vi "super small oscilloscope.vi"() -> ()   [LabVIEW 2017]
uses:
  <vilib>/Instr/_visa.llb/VISA Set IO Buffer Mask.ctl
  typedefs/reading3.ctl
  <vilib>/Platform/TimedLoop/XDataNode/timing_clust.ctl
  <vilib>/Platform/TimedLoop/XDataNode/nitl_modes.ctl
  <vilib>/Platform/TimedLoop/XDataNode/wakeup.ctl
  typedefs/reading1.ctl
  <vilib>/Analysis/6fits.llb/Curve Fitting Criteria.ctl
  <vilib>/Analysis/baseanly.llb/Mean (DBL).vi
  <vilib>/Instr/_visa.llb/VISA Configure Serial Port (Instr).vi
  <vilib>/platform/TimedLoop/XDataNode/XDataNode.xnode
  <vilib>/Platform/TimedLoop/XDataNode/XDNodeRunTimeDep.lvlib
  <vilib>/Analysis/NI_AALPro.lvlib
  <vilib>/ptbypt/NI_PtbyPt.lvlib
  <vilib>/Analysis/NI_AALBase.lvlib
panel:
  out "z accel":dbl format="%0.2f"
  out "Yaccel":dbl(slide) scale=-1.0..1.0
  out "Xaccel":dbl(slide) scale=-1.0..1.0
  in  "rest":bool
  out "error":i32
  out "deg/hr":dbl format="%0.2f"
  out "Waveform Chart":dbl(graph)
  out "angle":dbl
  out "slope":dbl
  out "magnet":cluster{dbl[], "Best Linear Fit":dbl[]}[](graph)
  in  "time range (s)":dbl=2.2 format="%#_13g"
  in  "stop 2":bool
  out "voltage":cluster{dbl[], dbl[]}[](graph)
  in  "update (ms)":i64=100
  out "error out":errorcluster
  in  "stop":bool
  in  "VISA resource name":refnum<visa-resource-name>
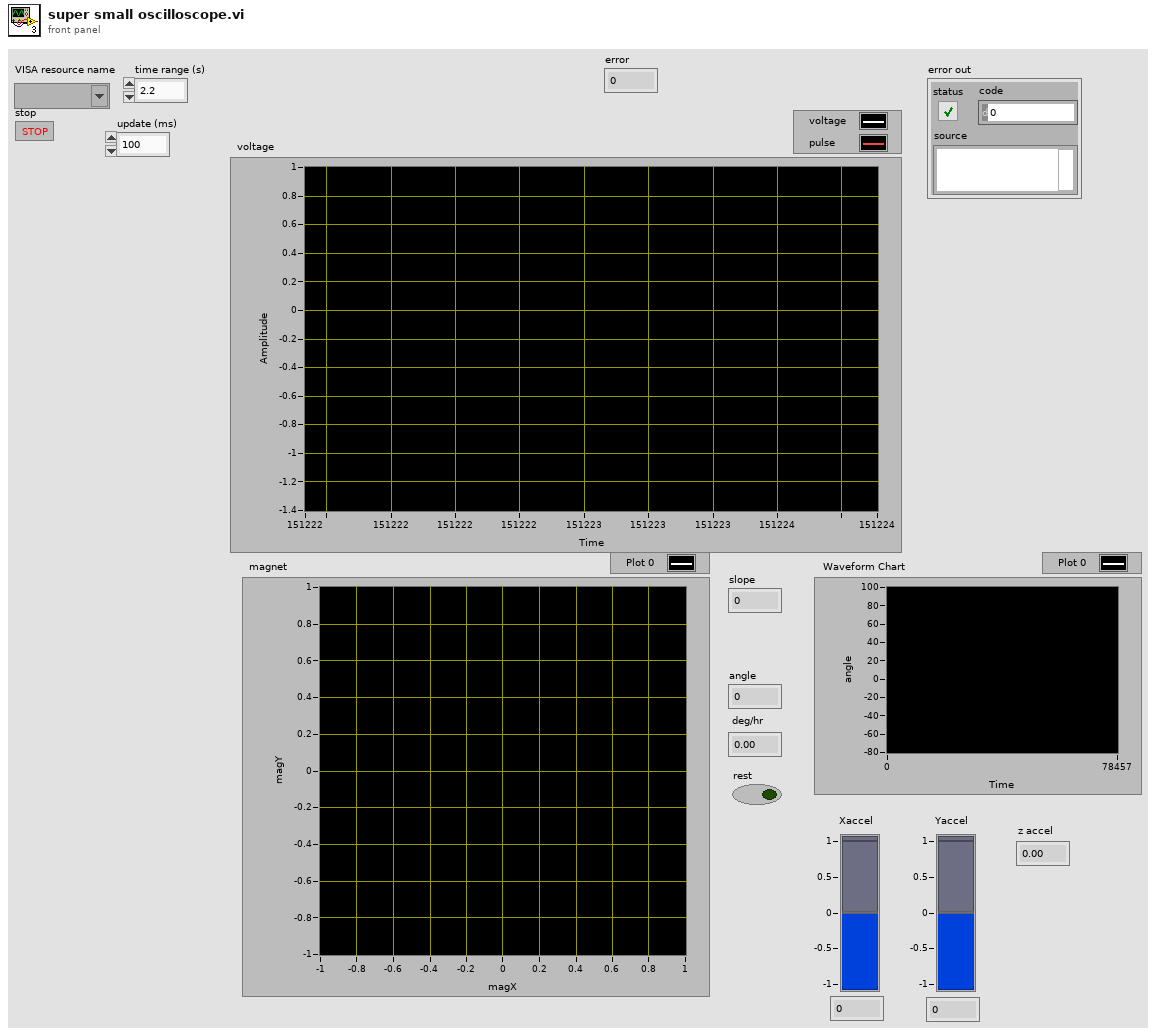
[diagram p1: front panel]
types:
  T1 = typedef "reading3.ctl" = cluster{"time":dbl, "x":dbl, "y":dbl, "z":dbl}
  T2 = typedef "VISA Set IO Buffer Mask.ctl" = u16
  T3 = typedef "reading1.ctl" = cluster{"time":dbl, "x":dbl}
  T4 = typedef "XDNodeRunTimeDep.lvlib/timing_clust.ctl" = cluster{"Expected End [f-1]":u64, "Actual End [f-1]":u64, "Finished Late? [f-1]":bool, "Expected End [i-1]":u64, "Actual End [i-1]":u64, "Finished Late? [i-1]":bool, "Expected Start [i]":u64, "Actual Start [i]":u64, "Expected Start [f]":u64, "Actual Start [f]":u64, "Source Name":string, "Structure Name":string, "Period":i64, "Deadline":i64, "Offset":i64, "Start":i64, "Priority":i32, "Timeout":i32, "Mode":T5, "Wakeup Reason":T6, "Error":errorcluster, "Source Type":string, "Secondary Source Type":string, "Global End Time":u64, "Global Start Time":u64, "Frame Duration":u64, "Iteration Duration":u64, "Assigned CPU":i32, "I/O Scan Engine Mode":u32}
  T5 = typedef "XDNodeRunTimeDep.lvlib/nitl_modes.ctl" = enum32{"No Change", "Process missed periods, maintain original phase", "Discard missed periods, maintain original phase", "Process missed periods, ignore original phase", "Discard missed periods, ignore original phase"}
  T6 = typedef "XDNodeRunTimeDep.lvlib/wakeup.ctl" = enum32{"Normal", "Aborted", "Asynchronous wakeup", "Timing source error", "Timed loop error", "Timeout"}
  T7 = typedef "NI_AALPro.lvlib/Curve Fitting Criteria.ctl" = u16
  T8 = cluster{"Best Linear Fit":dbl[], "Best Linear Fit":dbl[]}
  T9 = cluster{"Best Linear Fit":dbl[], "Best Linear Fit":dbl[]}[]
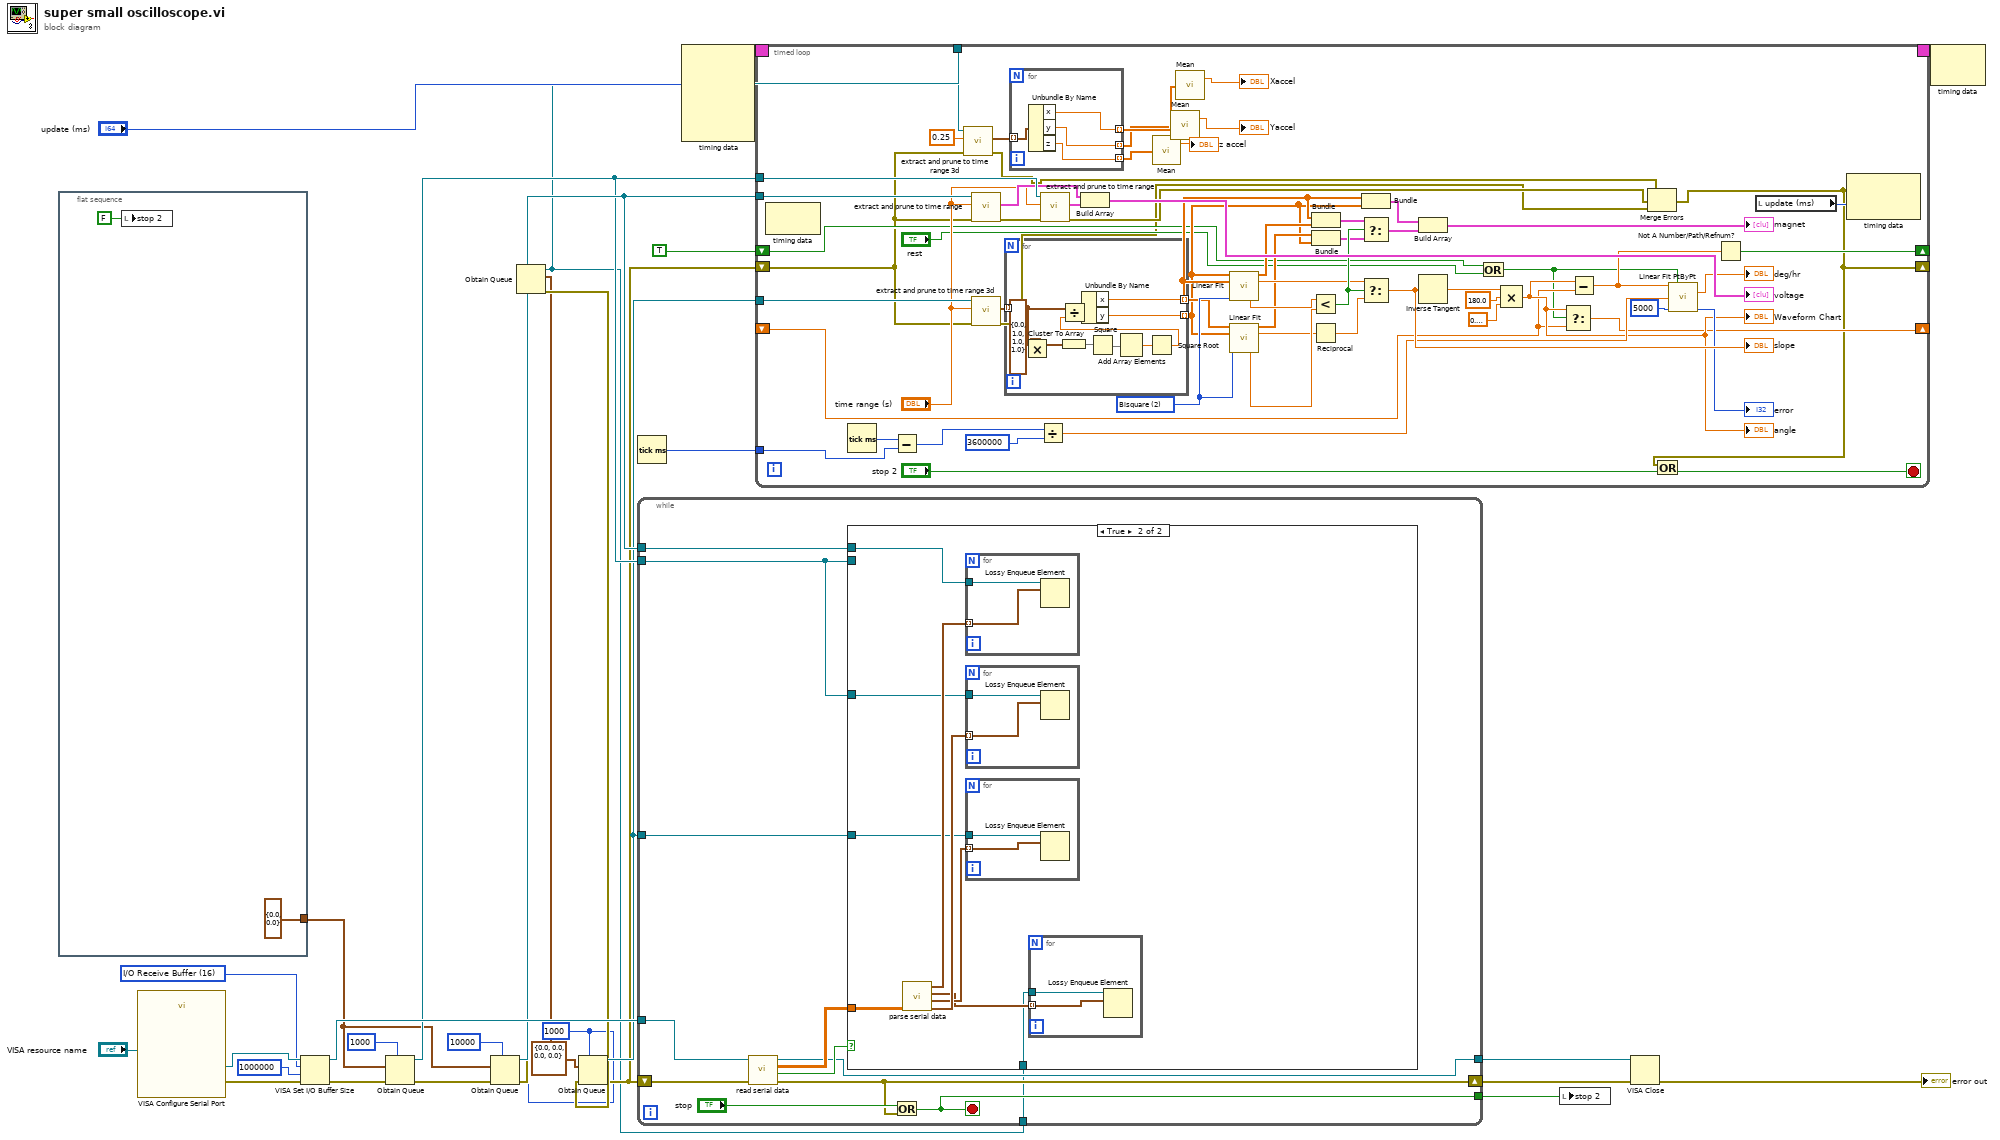
[diagram p0: block diagram]
diagram:
  w2 = 1000 ("max queue size (-1, unlimited)")
  w3 = T1 {"time"=0.0, "x"=0.0, "y"=0.0, "z"=0.0} ("reading3")
  w25 = T2 16 items=["I/O Receive Buffer"=16, "I/O Transmit Buffer"=32, "I/O Receive and Transmit Buffer"=48] ("Mask")
  n1 = flat-sequence {
    tunnel: [T3 {"time"=0.0, "x"=0.0} ("reading1")] -> w14
    frame #0 {
      n2 = local write "stop 2"(FALSE ("stop 2")) -> ()
    }
  }
  n3 = call-poly "VISA Configure Serial Port"("VISA resource name"="VISA resource name") -> ("VISA resource name out"=w28:refnum<visa-resource-name>, "error out"=w24:errorcluster)  [unwired: 13 in]
  n4 = VISA Set I/O Buffer Size(VISA resource name=w28, mask (16)=w25, size (4096)=u32 1000000, error in (no error)=w24) -> (VISA resource name out=w27:refnum<visa-resource-name>, error out=w17:errorcluster)
  n5 = Obtain Queue(max queue size (-1, unlimited)=1000, element data type=w14, error in (no error)=w17) -> (queue out=w15:refnum<queue>, error out=w13:errorcluster)  [unwired: 2 in, 1 out]
  n6 = Obtain Queue(max queue size (-1, unlimited)=10000, element data type=w14, error in (no error)=w13) -> (queue out=w19:refnum<queue>, error out=w6:errorcluster)  [unwired: 2 in, 1 out]
  n7 = Obtain Queue(max queue size (-1, unlimited)=w2, element data type=w3, error in (no error)=w6) -> (queue out=w1:refnum<queue>, error out=w5:errorcluster)  [unwired: 2 in, 1 out]
  n8 = Obtain Queue(max queue size (-1, unlimited)=w2, element data type=w3, error in (no error)=w5) -> (queue out=w9:refnum<queue>, error out=w4:errorcluster)  [unwired: 2 in, 1 out]
  n9 = Tick Count (ms)() -> (millisecond timer value=w8:u32)
  n10 = while {
    tunnel: w27 -> [w42]
    shift-right: [w38] -> w11
    shift-left: w4 -> [w41]
    tunnel: w19 -> [w37]
    tunnel: [w36] -> w18
    tunnel: w15 -> [w35]
    tunnel: [w34] -> w12
    tunnel: w9 -> [w33]
    tunnel: w1 -> [w32]
    stop <- w36 stop-if-true
    n11 = call "read serial data.vi"("error in (no error)"=w41, "serial port"=w42) -> ("error out"=w38:errorcluster, "data read"=w39:bool, "serial data"=w40:dbl[][], "VISA resource name out"=w34:refnum<visa-resource-name>)  [unwired: 6 in]
    n12 = case shown="True" w39 {
      tunnel: w40 -> [_ w52]
      tunnel: w37 -> [_ w50]
      tunnel: w35 -> [_ _]
      tunnel: w35 -> [_ w49]
      tunnel: w33 -> [_ w46]
      tunnel: w32 -> [_ w44]
      frame False {
      }
      frame True {
        n13 = call "parse serial data.vi"("serial data"=w52) -> ("coil data"=w48:T3[], "mag data"=w47:T1[], "accel data"=w45:T1[], "voltage data"=w51:T3[])  [unwired: 7 in]
        n14 = for {
          tunnel: w51 -> [w59] mode=indexing
          tunnel: w50 -> [w60]
          n15 = Lossy Enqueue Element(queue=w60, element=w59) -> ()  [unwired: 1 in, 4 out]
        }
        n16 = for {
          tunnel: w49 -> [w58]
          tunnel: w48 -> [w57] mode=indexing
          n17 = Lossy Enqueue Element(queue=w58, element=w57) -> ()  [unwired: 1 in, 4 out]
        }
        n18 = for {
          tunnel: w47 -> [w56] mode=indexing
          tunnel: w46 -> [w55]
          n19 = Lossy Enqueue Element(queue=w55, element=w56) -> ()  [unwired: 1 in, 4 out]
        }
        n20 = for {
          tunnel: w45 -> [w54] mode=indexing
          tunnel: w44 -> [w53]
          n21 = Lossy Enqueue Element(queue=w53, element=w54) -> ()  [unwired: 1 in, 4 out]
        }
      }
    }
    n22 = Or(x="stop", y=w38) -> (x .or. y?=w36:bool)
  }
  n23 = node-c288("update (ms)") -> (w22:T4)  [unwired: 4 in]
  n24 = timed-loop {
    timing: w22 -> [_]
    timing-out: [_] -> w21
    tunnel: w19 -> [w119]
    tunnel: w15 -> [w117]
    tunnel: w9 -> [w114]
    tunnel: w8 -> [w89]
    shift-right: [w83] -> _
    shift-left: _ -> [w82]
    shift-right: [w80] -> _
    shift-left: TRUE -> [w79]
    shift-right: [w72] -> _
    shift-left: w4 -> [w62]
    tunnel: w1 -> [w70]
    stop <- w73 stop-if-true
    w105 = T7 2 items=["Least Square", "Least Absolute Residual", "Bisquare"] ("method")
    n25 = node-c288() -> ()  [unwired: 1 in, 1 out]
    n26 = Tick Count (ms)() -> (millisecond timer value=w90:u32)
    n27 = Subtract(x=w90, y=w89) -> (x-y=w88:u32)
    n28 = call "extract and prune to time range 3d.vi"("error in (no error)"=w62, "time range"=0.25, "queue in"=w70) -> ("error out"=w61:errorcluster, "pruned data"=w69:T1[])  [unwired: 6 in, 1 out]
    n29 = call "extract and prune to time range.vi"("error in (no error)"=w62, "time range"="time range (s)", "time and val queue"=w119) -> ("error out"=w118:errorcluster, "graph"=w115:cluster{dbl[], dbl[]})  [unwired: 6 in, 1 out]
    n30 = call "extract and prune to time range 3d.vi"("error in (no error)"=w62, "time range"="time range (s)", "queue in"=w114) -> ("error out"=w74:errorcluster, "pruned data"=w112:T1[])  [unwired: 6 in, 1 out]
    n31 = for {
      tunnel: w112 -> [w134] mode=indexing
      tunnel: [w136] -> w93 mode=indexing
      tunnel: [w135] -> w92 mode=indexing
      n32 = Multiply(x=w134, y=T1 {"time"=0.0, "x"=1.0, "y"=1.0, "z"=1.0}) -> (x*y=w128:T1)
      n33 = Cluster To Array(cluster=w128) -> (array=w133:dbl[])
      n34 = Square(x=w133) -> (x^2=w132:dbl[])
      n35 = Add Array Elements(numeric array=w132) -> (sum=w131:dbl)
      n36 = Square Root(x=w131) -> (sqrt(x)=w129:dbl)
      n37 = Divide(x=w134, y=w129) -> (x/y=w130:T1)
      n38 = Unbundle By Name(w130) -> ("x"=w136:dbl, "y"=w135:dbl)
    }
    n39 = for {
      tunnel: w69 -> [w126] mode=indexing
      tunnel: [w125] -> w68 mode=indexing
      tunnel: [w124] -> w67 mode=indexing
      tunnel: [w123] -> w64 mode=indexing
      n40 = Unbundle By Name(w126) -> ("x"=w125:dbl, "y"=w124:dbl, "z"=w123:dbl)
    }
    n41 = Divide(x=w88, y=u32 3600000) -> (x/y=w86:dbl)
    n42 = call "extract and prune to time range.vi"("error in (no error)"=w118, "time range"="time range (s)", "time and val queue"=w117) -> ("error out"=w75:errorcluster, "graph"=w116:cluster{dbl[], dbl[]})  [unwired: 6 in, 1 out]
    n43 = Build Array(w115, w116) -> (→"voltage":cluster{dbl[], dbl[]}[])
    n44 = call-poly <vilib>:"Mean.vi"("X"=w64) -> ("mean"=→"z accel":dbl)  [unwired: 1 out]
    n45 = call-poly <vilib>:"Mean.vi"("X"=w67) -> ("mean"=→"Yaccel":dbl)  [unwired: 1 out]
    n46 = call-poly <vilib>:"Mean.vi"("X"=w68) -> ("mean"=→"Xaccel":dbl)  [unwired: 1 out]
    n47 = call <vilib>:"Linear Fit.vi"("Y"=w92, "X"=w93, "method"=w105) -> ("Best Linear Fit"=w111:dbl[], "slope"=w99:dbl, "residue"=w103:dbl)  [unwired: 8 in, 2 out]
    n48 = call <vilib>:"Linear Fit.vi"("Y"=w93, "X"=w92, "method"=w105) -> ("Best Linear Fit"=w97:dbl[], "slope"=w95:dbl, "residue"=w104:dbl)  [unwired: 8 in, 2 out]
    n49 = Less?(x=w103, y=w104) -> (x < y?=w100:bool)
    n50 = Reciprocal(x=w95) -> (1/x=w94:dbl)
    n51 = Bundle(w93, "Best Linear Fit"=w111) -> (w102:cluster{dbl[], "Best Linear Fit":dbl[]})  [unwired: 1 in]
    n52 = Bundle("Best Linear Fit"=w97, w92) -> (w96:cluster{"Best Linear Fit":dbl[], dbl[]})  [unwired: 1 in]
    n53 = Bundle(w93, w92) -> (w110:cluster{dbl[], dbl[]})  [unwired: 1 in]
    n54 = Select(t=w102, s=w100, f=w96) -> (s? t:f=w101:T8)
    n55 = Select(t=w99, s=w100, f=w94) -> (s? t:f=w98:dbl)
    "slope" <- w98
    n56 = Build Array(w110, w101) -> (→"magnet":T9)
    n57 = Inverse Tangent(1:w98) -> (0:w108:dbl)
    n58 = Or(x=w79, y="rest") -> (x .or. y?=w77:bool)
    n59 = Compound Arithmetic op=MULTIPLY(w108, 180.0 ("y"), 0.3183098861837907) -> (w84:dbl)
    "angle" <- w84
    "Waveform Chart" <- w84
    n60 = Select(t=w84, s=w77, f=w82) -> (s? t:f=w83:dbl)
    n61 = Subtract(x=w84, y=w82) -> (x-y=w78:dbl)
    n62 = Merge Errors(w61, w75, w74) -> (w72:errorcluster)
    n63 = Or(x=w72, y="stop 2") -> (x .or. y?=w73:bool)
    n64 = call <vilib>:"Linear Fit PtByPt.vi"("y"=w78, "initialize"=w77, "x"=w86, "sample length"=5000) -> ("slope"=→"deg/hr":dbl, "error"=→"error":i32)  [unwired: 7 in, 3 out]
    n65 = Not A Number/Path/Refnum?(number/path/refnum=w78) -> (NaN/Path/Refnum?=w80:bool)
    n66 = local read "update (ms)"() -> (w122:i64)
    n67 = node-c288(w72, w122) -> ()  [unwired: 1 out]
  }
  n68 = local write "stop 2"(w18) -> ()
  n69 = VISA Close(VISA resource name=w12, error in (no error)=w11) -> (error out=→"error out":errorcluster)
  n70 = node-c288(w21) -> ()  [unwired: 1 out]
